vi "Test_PublishUnnamedDbl_DoNotPublish_ReturnError.vi"(8 "error in (no error)":errorcluster, 11 "TestCase in":refnum<class "TestModelPublishAndObserve.lvclass">) -> (0 "error out":errorcluster, 3 "TestCase out":refnum<class "TestModelPublishAndObserve.lvclass">)   [LabVIEW 2020, in "TestModelPublishAndObserve.lvclass"]
uses:
  TestModelPublishAndObserve.lvclass
  TestModelPublishAndObserve.lvclass/TestModelPublishAndObserve.ctl
  24bf8875-c008-4f22-9bfa-88e42476d167.vi
  <vilib>/ActorFramework/Actor/Actor.lvclass
  Source/Mediator/Mediator/Mediator.lvclass
  <vilib>/ActorFramework/Stop Msg/Stop Msg.lvclass
  Doubles/RootModelPublishesDoubleFloat/RootModelPublishesDoubleFloat.lvclass
  C:/Git/mva-core/Source/RootModel/RootModel/RootModel.lvclass
  C:/Git/mva-core/Source/IModel/IModel/IModel.lvclass
  C:/Git/mva-core/Source/IObserver/IObserver/IObserver.lvclass
  C:/Program Files (x86)/National Instruments/LabVIEW 2020/vi.lib/ActorFramework/Actor/Actor.lvclass
  C:/Git/mva-core/Test/Doubles/RootModelPublishesDoubleFloat/RootModelPublishesDoubleFloat.lvclass
panel:
  out "Return Error":errorcluster
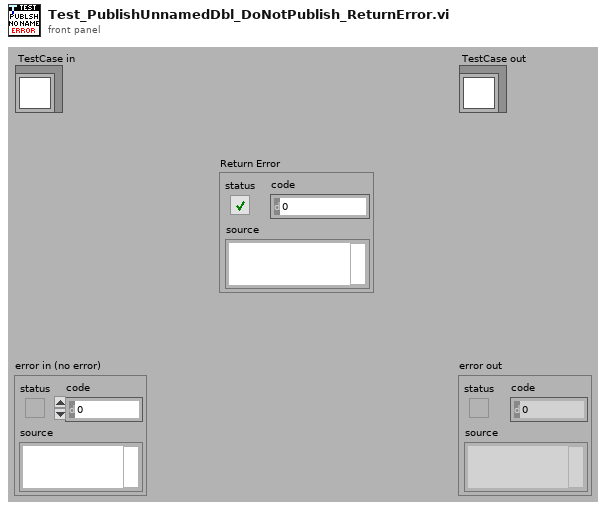
[diagram p1: front panel]
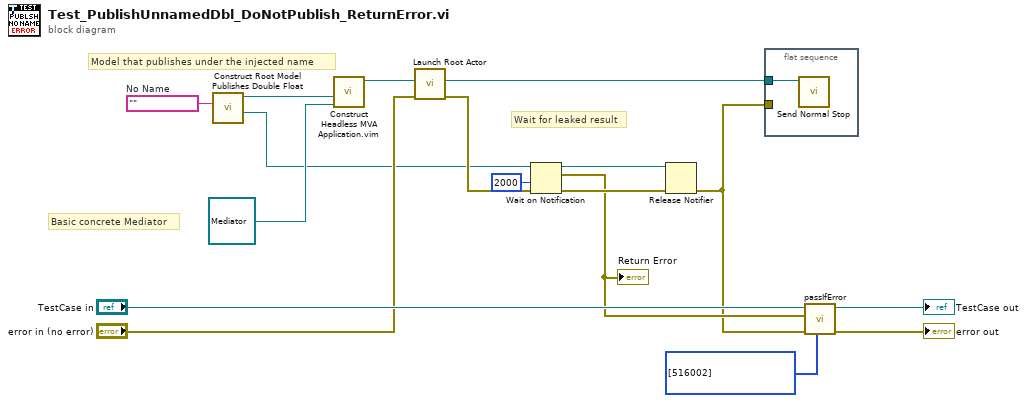
[diagram p0: block diagram]
diagram:
  w1 = ""  # No Name
  # "Model that publishes under the injected name"
  # "Wait for leaked result"
  # "Basic concrete Mediator"
  n1 = call "Construct Root Model Publishes Double Float.vi"("Datum Name"=w1) -> ("Error Notifier"=w3:refnum<notifier>, "RootModelPublishesDoubleFloat out"=w4:refnum<class "RootModelPublishesDoubleFloat.lvclass">)  [unwired: 9 in]
  n2 = call "Construct Headless MVA Application.vim"("Mediator Type"=refnum<class "Mediator.lvclass"> refnum ("Mediator.lvlib:Mediator.lvclass"), "RootModel in"=w4) -> ("RootModel out"=w14:refnum<class "RootModelPublishesDoubleFloat.lvclass">)  [unwired: 9 in]
  n3 = call <vilib>:"Launch Root Actor.vi"("error in (no error)"="error in (no error)", "Actor"=w14) -> ("error out"=w9:errorcluster, "Actor's Enqueuer"=w7:refnum<class "Message Enqueuer.lvclass">)  [unwired: 8 in]
  n4 = Wait on Notification(notifier=w3, timeout in ms (-1)=2000, error in (no error)=w9) -> (notifier out=w13:refnum<notifier>, notification=w8:errorcluster, error out=w11:errorcluster)  [unwired: 1 in, 1 out]
  "Return Error" <- w8
  n5 = Release Notifier(notifier=w13, error in (no error)=w11) -> (error out=w6:errorcluster)  [unwired: 1 in, 2 out]
  n6 = flat-sequence {
    tunnel: w7 -> [w18]
    tunnel: w6 -> [_]
    frame #0 {
      n7 = call <vilib>:"Send Normal Stop.vi"("Message Enqueuer"=w18) -> ()  [unwired: 10 in, 1 out]
    }
  }
  n8 = call-dynamic "passIfError.vi"("passing error codes (default = any error code)"=i32[] [516002], "error in (no error)"=w6, "error"=w8, "TestCase in"="TestCase in") -> ("error out"=→"error out":errorcluster, "TestCase out"=→"TestCase out":refnum<class "TestModelPublishAndObserve.lvclass">)  [unwired: 6 in]
